vi "SRingStopThread.vi"   [LabVIEW 2015]
uses:
  TRANCON/DLL/lwlscdll.dll
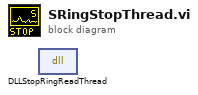
[diagram p0: block diagram]
diagram:
  n1 = dll-call lib="G:/SD/TRANCON/DLL/lwlscdll.dll" fn="DLLStopRingReadThread"() -> ()  [unwired: 4 in, 2 out]
